vi "UDP ROS Reciever.vi"(8 "error in (no error)":errorcluster, 9 "ENQUE DIRECTLY":refnum<queue>, 10 "milliseconds to wait":u32, 11 "UDP Network Connection in":refnum<k16>) -> (0 "error out":errorcluster)   [LabVIEW 2016]
uses:
  Globale Variablen VI/AutonomousMode.vi
  Globale Variablen VI/Global Variables.vi
  Globale Variablen VI/RadSensoren.vi
panel:
  out "data out":string
  out "vs recieved":dbl
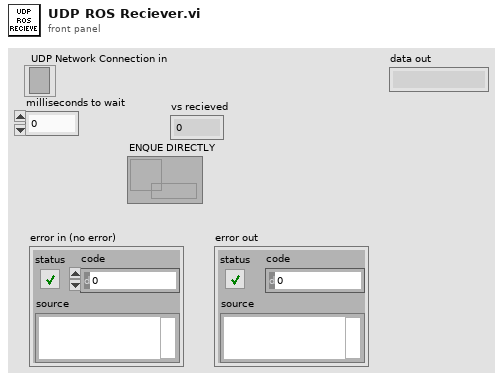
[diagram p1: front panel]
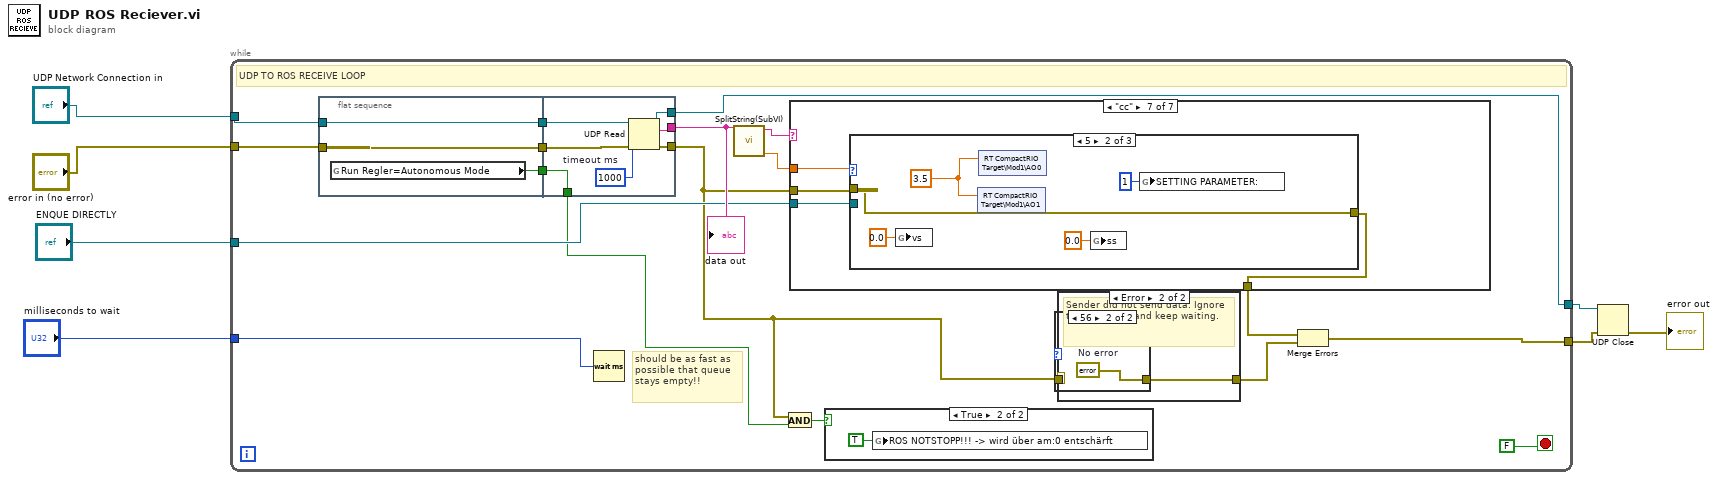
[diagram p0: block diagram]
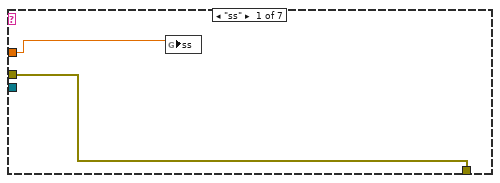
[diagram p3: hidden frame]
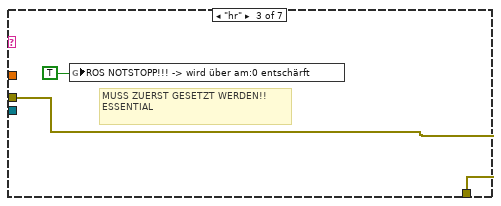
[diagram p5: hidden frame]
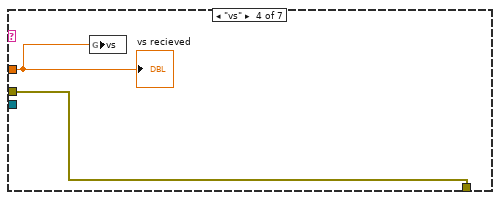
[diagram p6: hidden frame]
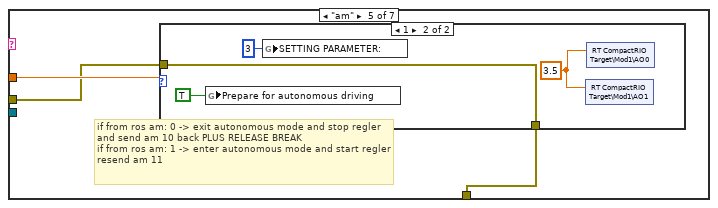
[diagram p7: hidden frame]
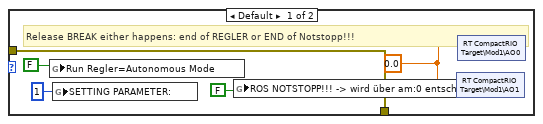
[diagram p8: hidden frame]
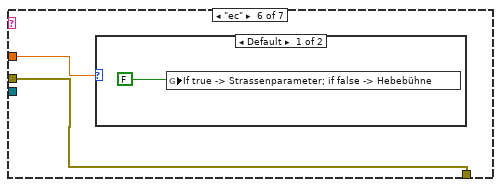
[diagram p9: hidden frame]
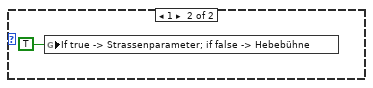
[diagram p10: hidden frame]
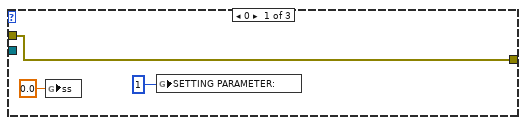
[diagram p11: hidden frame]
diagram:
  n1 = while {
    tunnel: [w23] -> w6
    tunnel: "UDP Network Connection in" -> [w25]
    tunnel: "error in (no error)" -> [w24]
    tunnel: "milliseconds to wait" -> [w19]
    tunnel: [w16] -> w2
    tunnel: "ENQUE DIRECTLY" -> [w15]
    stop <- FALSE stop-if-true
    # "should be as fast as possible that queue stays empty!!"
    # "UDP TO ROS RECEIVE LOOP"
    n2 = flat-sequence {
      tunnel: w24 -> [w27]
      tunnel: w25 -> [w28]
      tunnel: [w28] -> w11
      tunnel: [w27] -> w10
      tunnel: [w26] -> w8
      tunnel: [w32] -> w23
      tunnel: [w31] -> w20
      tunnel: [w30] -> w13
      tunnel: w11 -> [w34]
      tunnel: w10 -> [w33]
      tunnel: [w29] -> w9
      tunnel: w8 -> [w29]
      frame #0 {
        n3 = global read "AutonomousMode.vi" "Run Regler=Autonomous Mode"() -> (w26:bool)
      }
      frame #1 {
        w35 = 1000  # timeout ms
        n4 = UDP Read(connection ID=w34, timeout ms (25000)=w35, 8:w33) -> (data out=w31:string, error out=w30:errorcluster, 3:w32:refnum<k16>)  [unwired: 3 out]
      }
    }
    n5 = Wait (ms)(milliseconds to wait=w19) -> ()  [unwired: 1 out]
    n6 = call "SplitString(SubVI).vi"("data in"=w20) -> ("Numeric"=w22:dbl, "String 3"=w21:string)  [unwired: 9 in]
    n7 = And(x=w13, y=w9) -> (x .and. y?=w14:bool)
    n8 = case shown="\"cc\"" w21 {
      tunnel: w22 -> [w37 _ _ w43 w46 w57 w63]
      tunnel: w13 -> [w38 w39 w41 w42 w45 w56 w62]
      tunnel: [w38 w39 w41 w42 w44 w56 w61] -> w17
      tunnel: w15 -> [_ _ _ _ _ _ w60]
      frame "ss" {
        n9 = global write "Global Variables.vi" "ss"(w37) -> ()
      }
      frame Default {
      }
      frame "hr" {
        # "MUSS ZUERST GESETZT WERDEN!! ESSENTIAL"
        n10 = global write "AutonomousMode.vi" "ROS NOTSTOPP!!! -> wird über am:0 entschärft"(TRUE ("Run Regler=Autonomous Mode")) -> ()
      }
      frame "vs" {
        n11 = global write "RadSensoren.vi" "vs"(w43) -> ()
        "vs recieved" <- w43
      }
      frame "am" {
        # "if from ros am: 0 -> exit autonomous mode and stop regler and send am 10 back PLUS RELEASE BREAK\nif from ros am: 1 -> enter autonomous mode and start regler resend am 11"
        n12 = case shown="1" w46 {
          tunnel: w45 -> [w48 w55]
          tunnel: [w48 w55] -> w44
          frame Default {
            w47 = 0.0
            # "Release BREAK either happens: end of REGLER or END of Notstopp!!!"
            n13 = global write "AutonomousMode.vi" "Run Regler=Autonomous Mode"(FALSE ("Run Regler=Autonomous Mode")) -> ()
            n14 = global write "Global Variables.vi" "SETTING PARAMETER:"(1 ("SETTING PARAMETER:")) -> ()
            n15 = global write "AutonomousMode.vi" "ROS NOTSTOPP!!! -> wird über am:0 entschärft"(FALSE ("Run Regler=Autonomous Mode")) -> ()
            n16 = shared-variable "RT CompactRIO Target\\Mod1\\AO1"(w47) -> ()  [unwired: 1 in, 1 out]
            n17 = shared-variable "RT CompactRIO Target\\Mod1\\AO0"(w47) -> ()  [unwired: 1 in, 1 out]
          }
          frame 1 {
            w52 = 3.5
            n18 = global write "AutonomousMode.vi" "Prepare for autonomous driving"(TRUE) -> ()
            n19 = global write "Global Variables.vi" "SETTING PARAMETER:"(3 ("SETTING PARAMETER:")) -> ()
            n20 = shared-variable "RT CompactRIO Target\\Mod1\\AO1"(w52) -> ()  [unwired: 1 in, 1 out]
            n21 = shared-variable "RT CompactRIO Target\\Mod1\\AO0"(w52) -> ()  [unwired: 1 in, 1 out]
          }
        }
      }
      frame "ec" {
        n22 = case shown="Default" w57 {
          frame Default {
            n23 = global write "AutonomousMode.vi" "If true -> Strassenparameter; if false -> Hebebühne"(FALSE) -> ()
          }
          frame 1 {
            n24 = global write "AutonomousMode.vi" "If true -> Strassenparameter; if false -> Hebebühne"(TRUE) -> ()
          }
        }
      }
      frame "cc" {
        n25 = case shown="5" w63 {
          tunnel: w62 -> [w66 w71 w72]
          tunnel: [w66 w71 w72] -> w61
          tunnel: w60 -> [_ _ _]
          frame 0 {
            n26 = global write "Global Variables.vi" "ss"(0.0 ("ss")) -> ()
            n27 = global write "Global Variables.vi" "SETTING PARAMETER:"(1 ("SETTING PARAMETER:")) -> ()
          }
          frame 5 {
            w70 = 3.5
            n28 = global write "RadSensoren.vi" "vs"(0.0 ("vs")) -> ()
            n29 = shared-variable "RT CompactRIO Target\\Mod1\\AO1"(w70) -> ()  [unwired: 1 in, 1 out]
            n30 = shared-variable "RT CompactRIO Target\\Mod1\\AO0"(w70) -> ()  [unwired: 1 in, 1 out]
            n31 = global write "Global Variables.vi" "ss"(0.0 ("ss")) -> ()
            n32 = global write "Global Variables.vi" "SETTING PARAMETER:"(1 ("SETTING PARAMETER:")) -> ()
          }
          frame Default {
          }
        }
      }
    }
    n33 = case shown="True" w14 {
      frame False {
      }
      frame True {
        n34 = global write "AutonomousMode.vi" "ROS NOTSTOPP!!! -> wird über am:0 entschärft"(TRUE ("ROS NOTSTOPP!!! -> wird über am:0 entschärft")) -> ()
      }
    }
    n35 = case shown="Error" w13 {
      selector: w13 -> [w73 w75]
      tunnel: [w73 w74] -> w18
      frame No Error {
        # "Sender sent data. Update the chart value."
      }
      frame Error {
        # "Sender did not send data. Ignore timeout error and keep waiting."
        n36 = Unbundle By Name(w75) -> ("code"=w76:i32)
        n37 = case shown="56" w76 {
          tunnel: w75 -> [w77 _]
          tunnel: [w77 w78] -> w74
          frame Default {
          }
          frame 56 {
            w78 = errorcluster {"status"=FALSE, "code"=0, "source"=""}  # No error
          }
        }
      }
    }
    n38 = Merge Errors(w17, w18) -> (w16:errorcluster)
    "data out" <- w20
  }
  n39 = UDP Close(connection ID=w6, 8:w2) -> (error out=→"error out":errorcluster)  [unwired: 1 out]
